vi "load.vi"(8 "error in (no error)":errorcluster, 10 "Node":refnum<k20>, 11 "HP8662A_RF_Generator in":refnum<class "HP8662A_RF_Generator.lvclass">) -> (0 "error out":errorcluster, 2 "node out":refnum<k20>, 3 "HP8662A_RF_Generator out":refnum<class "HP8662A_RF_Generator.lvclass">)   [LabVIEW 2013, in "HP8662A_RF_Generator.lvclass"]
uses:
  HP8662A_RF_Generator.lvclass
  RF_Generator_settings.ctl
  HP8662A_RF_Generator.lvclass/HP8662A_RF_Generator.ctl
  <vilib>/xml/Close Reference(Node).vi
  <vilib>/xml/NI_XML.lvlib
  <resource>/objmgr/DOMUserDefRef.rc
  GPIB.lvclass
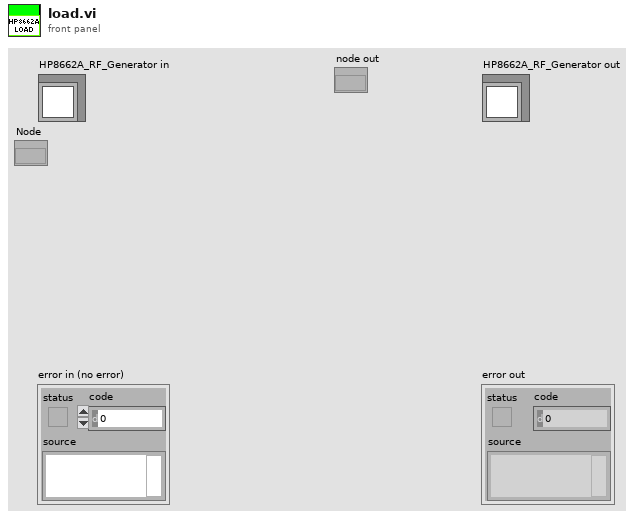
[diagram p1: front panel]
types:
  T1 = typedef "GPIB.lvclass/RF_Generator_settings.ctl" = cluster{"Enable":bool, "Description":string, "GPIB channel #":u8, "Frequency (MHz)":dbl, "Power (dBm)":dbl}
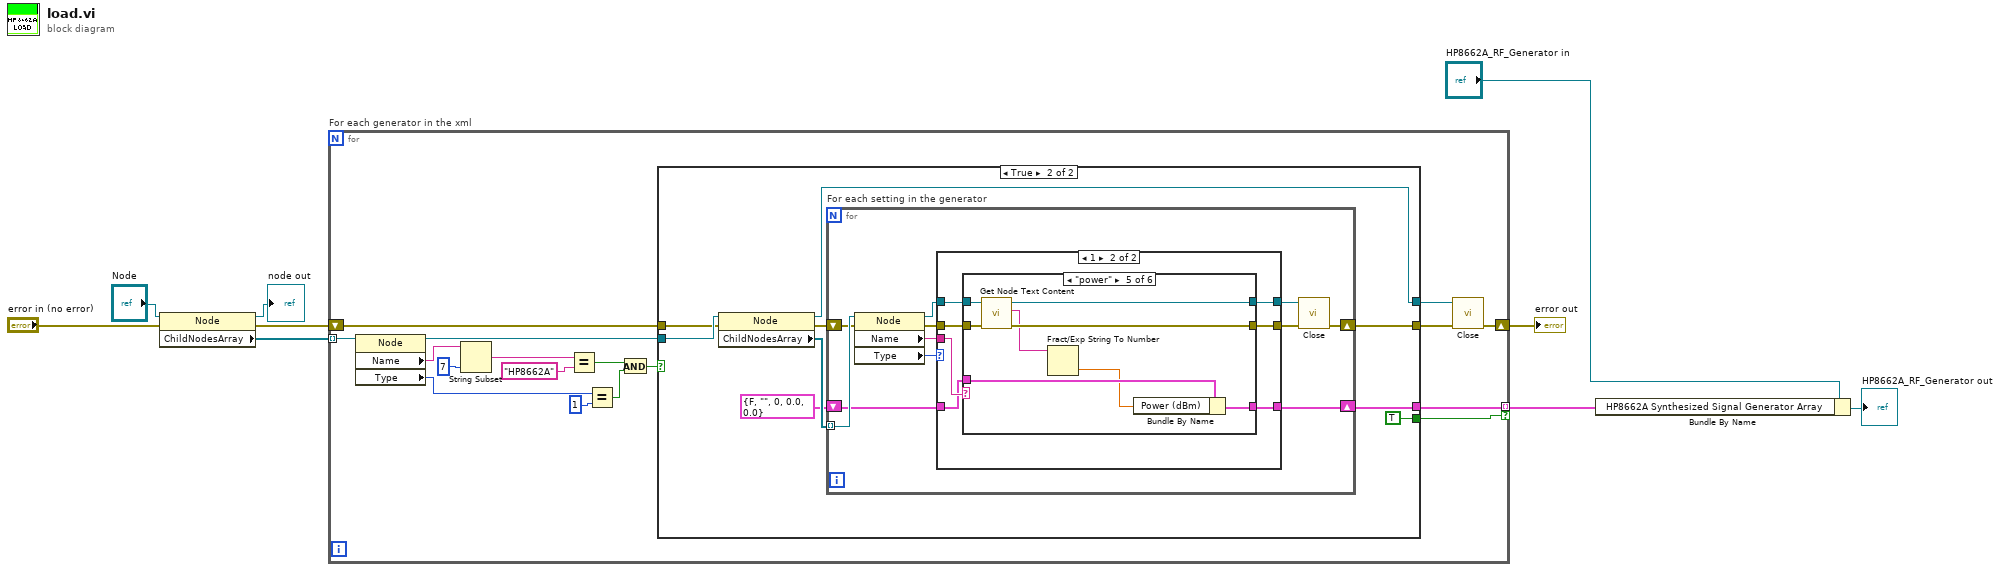
[diagram p0: block diagram]
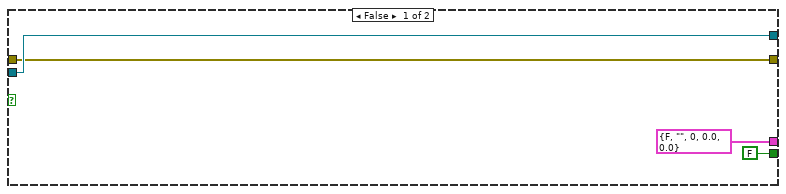
[diagram p2: hidden frame]
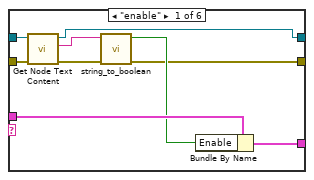
[diagram p4: hidden frame]
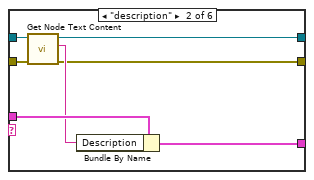
[diagram p5: hidden frame]
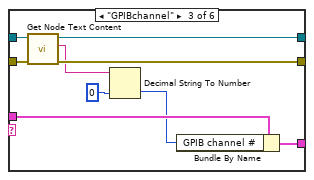
[diagram p6: hidden frame]
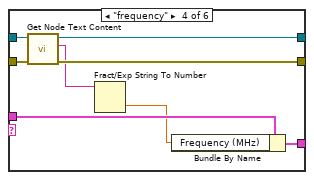
[diagram p7: hidden frame]
diagram:
  n1 = property class="Node"(reference="Node", error in="error in (no error)") -> (reference out=→"node out":refnum<k20>, error out=w1:errorcluster, "ChildNodesArray"=w2:refnum<k20>[])
  n2 = for "For each generator in the xml" {
    tunnel: w2 -> [w20] mode=indexing
    shift-right: [w23] -> w9
    shift-left: w1 -> [w26]
    tunnel: [w22] -> w6 mode=indexing if=w21
    n3 = property class="Node"(reference=w20) -> (reference out=w19:refnum<k20>, "Name"=w15:string, "Type"=w18:i32)  [unwired: 1 in, 1 out]
    n4 = String Subset(string=w15, length (rest)=7 ("length (rest)")) -> (substring=w13:string)  [unwired: 1 in]
    n5 = Equal?(x=w13, y="HP8662A") -> (x = y?=w11:bool)
    n6 = Equal?(x=w18, y=1) -> (x = y?=w16:bool)
    n7 = And(x=w11, y=w16) -> (x .and. y?=w10:bool)
    n8 = case shown="True" w10 {
      tunnel: w19 -> [w30 w39]
      tunnel: w26 -> [w29 w38]
      tunnel: [w30 w35] -> w25
      tunnel: [w29 w34] -> w24
      tunnel: [T1 {"Enable"=FALSE, "Description"="", "GPIB channel #"=0, "Frequency (MHz)"=0.0, "Power (dBm)"=0.0} ("Cluster") w33] -> w22
      tunnel: [FALSE TRUE] -> w21
      frame False {
      }
      frame True {
        n9 = property class="Node"(reference=w39, error in=w38) -> (reference out=w35:refnum<k20>, error out=w36:errorcluster, "ChildNodesArray"=w37:refnum<k20>[])
        n10 = for "For each setting in the generator" {
          shift-right: [w43] -> w34
          shift-left: w36 -> [w47]
          tunnel: w37 -> [w50] mode=indexing
          shift-right: [w41] -> w33
          shift-left: T1 {"Enable"=FALSE, "Description"="", "GPIB channel #"=0, "Frequency (MHz)"=0.0, "Power (dBm)"=0.0} ("Cluster") -> [w42]
          n11 = property class="Node"(reference=w50, error in=w47) -> (reference out=w45:refnum<k20>, error out=w48:errorcluster, "Name"=w49:string, "Type"=w40:i32)
          n12 = case shown="1" w40 {
            tunnel: w49 -> [_ w60]
            tunnel: w48 -> [w52 w59]
            tunnel: [w53 w58] -> w46
            tunnel: w45 -> [w53 w57]
            tunnel: [w52 w56] -> w44
            tunnel: w42 -> [w51 w55]
            tunnel: [w51 w54] -> w41
            frame Default {
            }
            frame 1 {
              n13 = case shown="\"power\"" w60 {
                tunnel: w59 -> [w68 w75 w84 w92 w100 w104]
                tunnel: [w61 w70 w80 w88 w96 w104] -> w56
                tunnel: [w65 w71 w81 w89 w97 w103] -> w58
                tunnel: w57 -> [w69 w76 w85 w93 w101 w103]
                tunnel: w55 -> [w67 w74 w83 w91 w99 w102]
                tunnel: [w66 w73 w82 w90 w98 w102] -> w54
                frame "enable" {
                  n14 = call <vilib>:"Get Node Text Content.vi"("error in (no error)"=w68, "node in"=w69) -> ("error out"=w62:errorcluster, "node text"=w64:string, "node out"=w65:refnum<k20>)  [unwired: 7 in]
                  n15 = call "string_to_boolean.vi"("error in"=w62, "string"=w64) -> ("error out"=w61:errorcluster, "boolean"=w63:bool)  [unwired: 8 in]
                  n16 = Bundle By Name(cluster=w67, "Enable"=w63) -> (w66:T1)
                }
                frame "description" {
                  n17 = call <vilib>:"Get Node Text Content.vi"("error in (no error)"=w75, "node in"=w76) -> ("error out"=w70:errorcluster, "node text"=w72:string, "node out"=w71:refnum<k20>)  [unwired: 7 in]
                  n18 = Bundle By Name(cluster=w74, "Description"=w72) -> (w73:T1)
                }
                frame "GPIBchannel" {
                  n19 = call <vilib>:"Get Node Text Content.vi"("error in (no error)"=w84, "node in"=w85) -> ("error out"=w80:errorcluster, "node text"=w79:string, "node out"=w81:refnum<k20>)  [unwired: 7 in]
                  n20 = Decimal String To Number(string=w79, default (0L)=u8 0 ("default (0 I32)")) -> (number=w78:u8)  [unwired: 1 in, 1 out]
                  n21 = Bundle By Name(cluster=w83, "GPIB channel #"=w78) -> (w82:T1)
                }
                frame "frequency" {
                  n22 = call <vilib>:"Get Node Text Content.vi"("error in (no error)"=w92, "node in"=w93) -> ("error out"=w88:errorcluster, "node text"=w87:string, "node out"=w89:refnum<k20>)  [unwired: 7 in]
                  n23 = Fract/Exp String To Number(string=w87) -> (number=w86:dbl)  [unwired: 3 in, 1 out]
                  n24 = Bundle By Name(cluster=w91, "Frequency (MHz)"=w86) -> (w90:T1)
                }
                frame "power" {
                  n25 = call <vilib>:"Get Node Text Content.vi"("error in (no error)"=w100, "node in"=w101) -> ("error out"=w96:errorcluster, "node text"=w95:string, "node out"=w97:refnum<k20>)  [unwired: 7 in]
                  n26 = Fract/Exp String To Number(string=w95) -> (number=w94:dbl)  [unwired: 3 in, 1 out]
                  n27 = Bundle By Name(cluster=w99, "Power (dBm)"=w94) -> (w98:T1)
                }
                frame Default {
                }
              }
            }
          }
          n28 = call-poly <vilib>:"Close.vi"("error in (no error)"=w44, "node"=w46) -> ("error out"=w43:errorcluster)  [unwired: 7 in]
        }
      }
    }
    n29 = call-poly <vilib>:"Close.vi"("error in (no error)"=w24, "node"=w25) -> ("error out"=w23:errorcluster)  [unwired: 7 in]
  }
  "error out" <- w9
  n30 = Bundle By Name(cluster="HP8662A_RF_Generator in", "HP8662A Synthesized Signal Generator Array"=w6) -> (→"HP8662A_RF_Generator out":refnum<class "HP8662A_RF_Generator.lvclass">)
